vi "GetAllClassesInProject.vi"(5 "error in (no error)":errorcluster) -> (15 "full class names":string[](array[string]), 16 "class paths":path[](array[path]), 17 "no active project?":bool, 19 "error out":errorcluster)   [LabVIEW 2017, in "G#RemoteProxy.lvclass"]
doc: "Returns all classes in the active project."
uses:
  G#RemoteProxy.lvclass
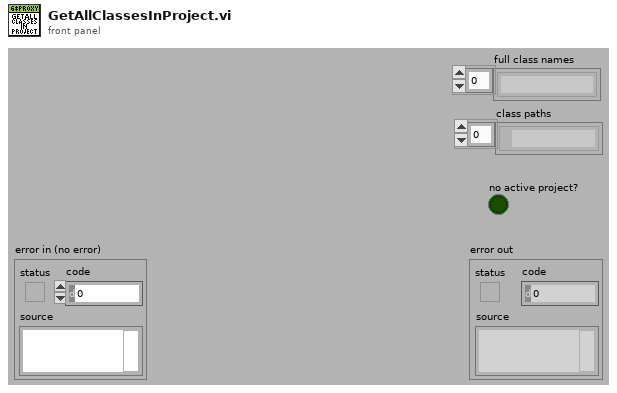
[diagram p1: front panel]
types:
  T1 = typedef "G#RemoteProxy.lvclass/ClassAttributesRef.ctl" = refnum<data-value>
  T2 = typedef "G#RemoteProxy.lvclass/ClassAttributesProxy.ctl" = cluster{"NoActiveProject":bool, "FullClassNames":string[], "FullClassPaths":path[], "RemoteRefs":refnum<class "G#Object.lvclass">[], "ProxyRefs":refnum<class "G#RemoteProxy.lvclass">[], "RemoteClassName":string[], "ProxyClassRefs":refnum<class "G#RemoteProxy.lvclass">[]}
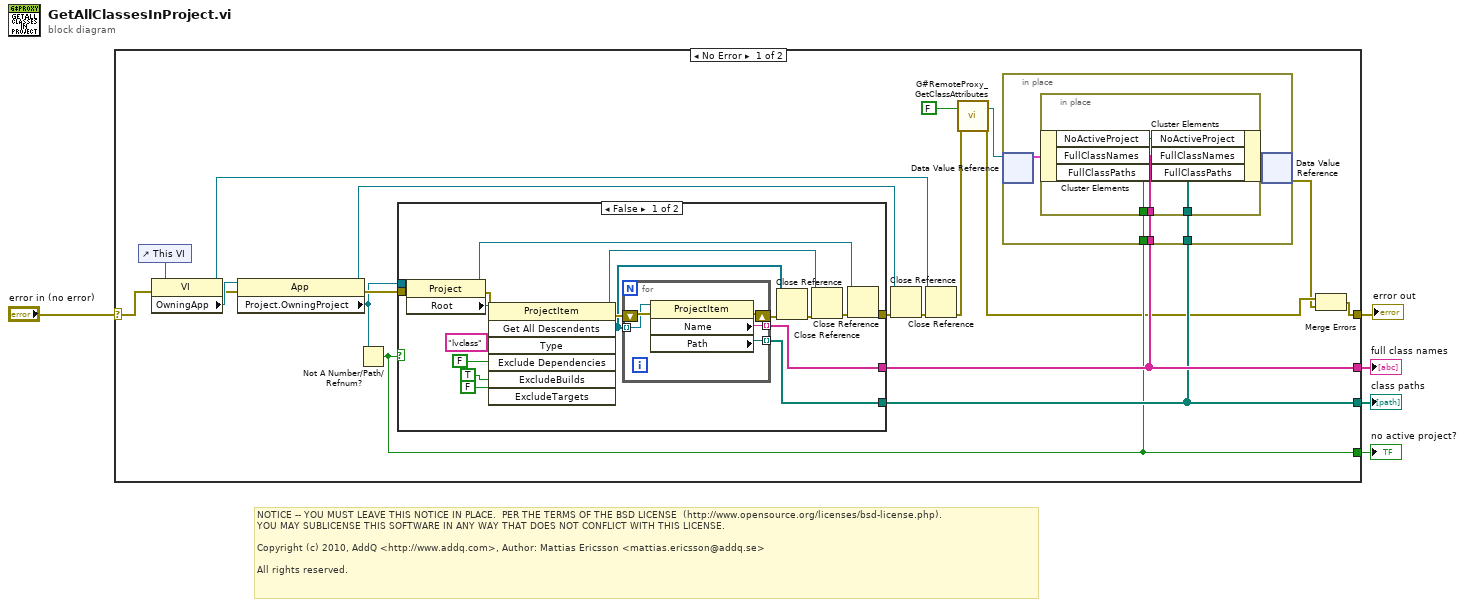
[diagram p0: block diagram]
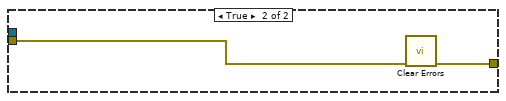
[diagram p2: hidden frame]
diagram:
  # "NOTICE -- YOU MUST LEAVE THIS NOTICE IN PLACE.  PER THE TERMS OF THE BSD LICENSE  (http://www.opensource.org/licenses/bsd-license.php).\nYOU MAY SUBLICENSE THIS SOFTWARE IN ANY WAY THAT DOES NOT CONFLICT WITH THIS LICENSE.\n\nCopyright (c) 2010, AddQ <http://www.addq.com>, Author: Mattias Ericsson <mattias.ericsson@addq.se>\n\nAll rights reserved."
  n1 = case shown="No Error" "error in (no error)" {
    selector: "error in (no error)" -> [w20 w58]
    tunnel: [w8 w58] -> w4
    tunnel: [w10 _] -> w2
    tunnel: [w11 _] -> w3
    tunnel: [w9 _] -> w1
    frame No Error {
      n2 = control-ref of="This VI"() -> (w19:refnum<vi>)
      n3 = property class="VI"(reference=w19, error in=w20) -> (reference out=w15:refnum<vi>, error out=w23:errorcluster, "OwningApp"=w24:refnum<vi>)
      n4 = property class="App"(reference=w24, error in=w23) -> (reference out=w16:refnum<vi>, error out=w22:errorcluster, "Project.OwningProject"=w21:refnum<vi>)
      n5 = Not A Number/Path/Refnum?(number/path/refnum=w21) -> (NaN/Path/Refnum?=w9:bool)
      n6 = case shown="False" w9 {
        tunnel: w22 -> [w50 w57]
        tunnel: w21 -> [w49 _]
        tunnel: [w36 w56] -> w17
        tunnel: [w35 _] -> w10
        tunnel: [w34 _] -> w11
        frame False {
          n7 = property class="Project"(reference=w49, error in=w50) -> (reference out=w37:refnum<vi>, error out=w46:errorcluster, "Root"=w48:refnum<vi>)
          n8 = invoke class="ProjectItem" method="Get All Descendents"(reference=w48, error in=w46, "Type"="lvclass", "Exclude Dependencies"=FALSE ("ExcludeDependencies"), "ExcludeBuilds"=TRUE ("ExcludeTargets"), "ExcludeTargets"=FALSE) -> (reference out=w44:refnum<vi>, error out=w45:errorcluster, "All Descendents"=w43:refnum<vi>[])  [unwired: 1 in, 4 out]
          n9 = for {
            shift-right: [w53] -> w40
            shift-left: w45 -> [w55]
            tunnel: w43 -> [w54] mode=indexing
            tunnel: [w52] -> w35 mode=indexing
            tunnel: [w51] -> w34 mode=indexing
            n10 = property class="ProjectItem"(reference=w54, error in=w55) -> (error out=w53:errorcluster, "Name"=w51:string, "Path"=w52:path)  [unwired: 1 out]
          }
          n11 = Close Reference(reference=w43, error in (no error)=w40) -> (error out=w39:errorcluster)
          n12 = Close Reference(reference=w44, error in (no error)=w39) -> (error out=w38:errorcluster)
          n13 = Close Reference(reference=w37, error in (no error)=w38) -> (error out=w36:errorcluster)
        }
        frame True {
          n14 = call <vilib>:"Clear Errors.vi"("error in (no error)"=w57) -> ("error out"=w56:errorcluster)  [unwired: 5 in, 1 out]
        }
      }
      n15 = Close Reference(reference=w16, error in (no error)=w17) -> (error out=w18:errorcluster)
      n16 = Close Reference(reference=w15, error in (no error)=w18) -> (error out=w14:errorcluster)
      n17 = call "G#RemoteProxy_GetClassAttributes.vi"("return data? (T)"=FALSE, "error in (no error)"=w14) -> ("class attributes ref"=w12:T1, "error out"=w7:errorcluster)  [unwired: 14 in, 2 out]
      n18 = in-place {
        in-place-border: w11 -> [w27]
        in-place-border: w10 -> [w26]
        in-place-border: w9 -> [w25]
        n19 = in-place-dvr #1(w12) -> (w28:T2)  [unwired: 1 out]
        n20 = in-place {
          in-place-border: w27 -> [w32]
          in-place-border: w26 -> [w31]
          in-place-border: w25 -> [w30]
          n21 = in-place-cluster #2(w28) -> ()  [unwired: 3 out]
          n22 = in-place-cluster #2("NoActiveProject"=w30, "FullClassNames"=w32, "FullClassPaths"=w31) -> (w29:T2)
        }
        n23 = in-place-dvr #1(w29) -> (w6:errorcluster)  [unwired: 1 out]
      }
      n24 = Merge Errors(w7, w6) -> (w8:errorcluster)
    }
    frame Error {
    }
  }
  "error out" <- w4
  "full class names" <- w3
  "class paths" <- w2
  "no active project?" <- w1
